vi "串口设备参数设置.vi"(8 "布尔文本.文本":string, 9 "section (optional)":string, 10 "监测项描述":string) -> (2 "布尔":bool=TRUE, 3 "输出簇":T1={"监测项描述:输出"="", "连接方式"=enum."串口", "端口"="", "IP address:"="", "Port:"="", "站号"=19200, "传感器型号"="", "波特率"=19200, "data bits"=8, "停止位"=10, "奇偶校验"=0} {"data bits" min=5 max=8 step=1; "停止位" items=["1.0"=10, "1.5"=15, "2.0"=20]; "奇偶校验" items=["None", "Odd", "Even", "Mark", "Space"]})   [LabVIEW 2016, in "环境动力监测库.lvlib"]
uses:
  <vilib>/Utility/miscctls.llb/LVPointTypeDef.ctl
  <vilib>/Utility/config.llb/NI_LVConfig.lvlib
panel:
  in  "参数配置":bool
  in  "连接方式:":enum16{"串口", "TCP"}(ring)
  in  "IP address:":string
  in  "Port:":string
  in  "data bits":u64=8 caption="数据比特" min=5 max=8 step=1
  in  "波特率":u64=19200
  in  "停止位":u16(ring)=10 items=["1.0"=10, "1.5"=15, "2.0"=20]
  in  "奇偶校验":u16(ring) items=["None", "Odd", "Even", "Mark", "Space"]
  in  "传感器型号:":string(combo)
  in  "输入簇":T1={"监测项描述:输出"="", "连接方式"=enum."串口", "端口"="", "IP address:"="", "Port:"="", "站号"=19200, "传感器型号"="", "波特率"=19200, "data bits"=8, "停止位"=10, "奇偶校验"=0} {"data bits" min=5 max=8 step=1; "停止位" items=["1.0"=10, "1.5"=15, "2.0"=20]; "奇偶校验" items=["None", "Odd", "Even", "Mark", "Space"]}
  in  "站号":u64
  in  "返回":bool
  in  "增加":bool
  in  "端口:":T2(ring)
  in  "监测项描述:":string
  # "基本设置"
  # "如:红外XX"
  # "传感器选择"
  # "端口选择"
  # "站号配置"
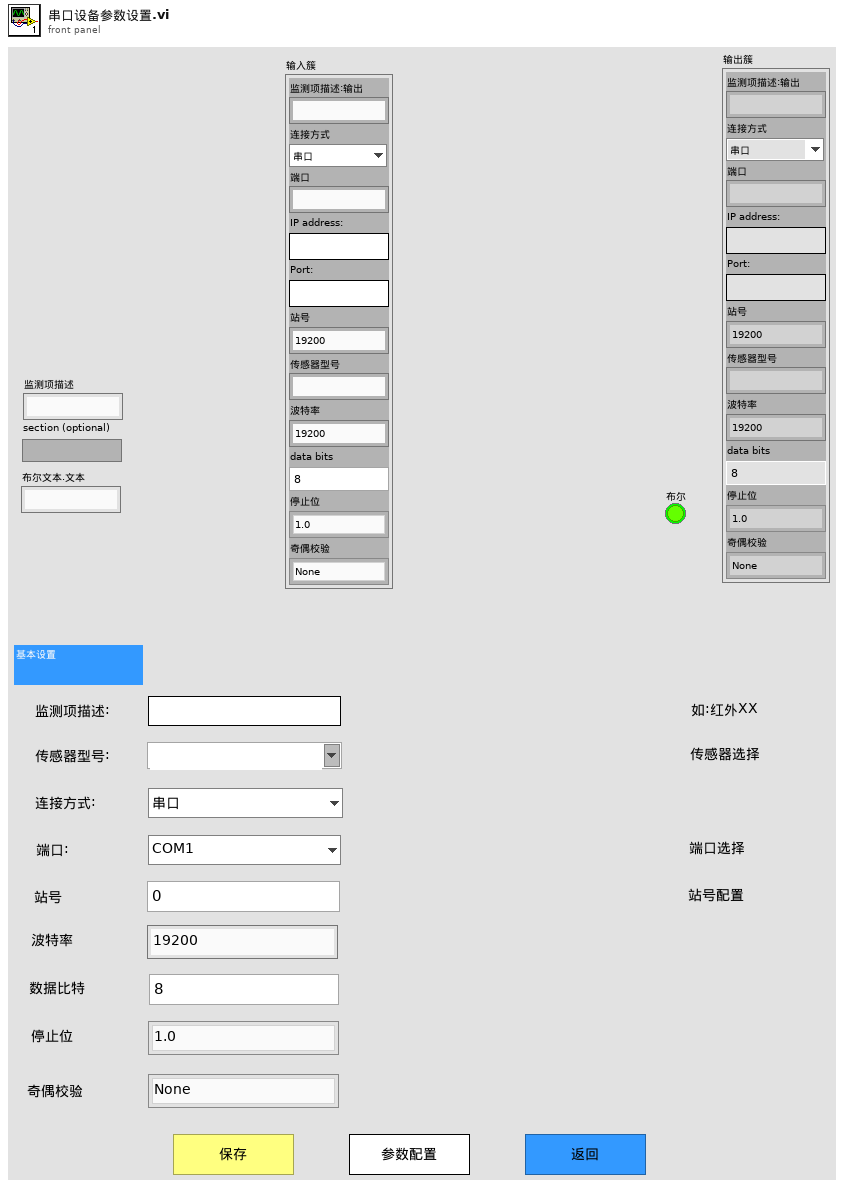
[diagram p1: front panel]
types:
  T1 = cluster{"监测项描述:输出":string, "连接方式":enum16{"串口", "TCP"}, "端口":string, "IP address:":string, "Port:":string, "站号":u64, "传感器型号":string, "波特率":u64, "data bits":u64, "停止位":u16, "奇偶校验":u16}
  T2 = enum16{"COM1", "COM2", "COM3", "COM4", "COM5", "COM6", "COM7", "COM8", "COM9", "COM10", "COM11", "COM12", "COM13", "COM14", "COM15", "COM16", "COM17", "COM18", "COM19", "COM20"}
  T3 = typedef "LVPointTypeDef.ctl" = cluster{"Horizontal":i16, "Vertical":i16}
  T4 = typedef "NI_LVConfig.lvlib/Config Data RefNum.ctl" = refnum<k1>
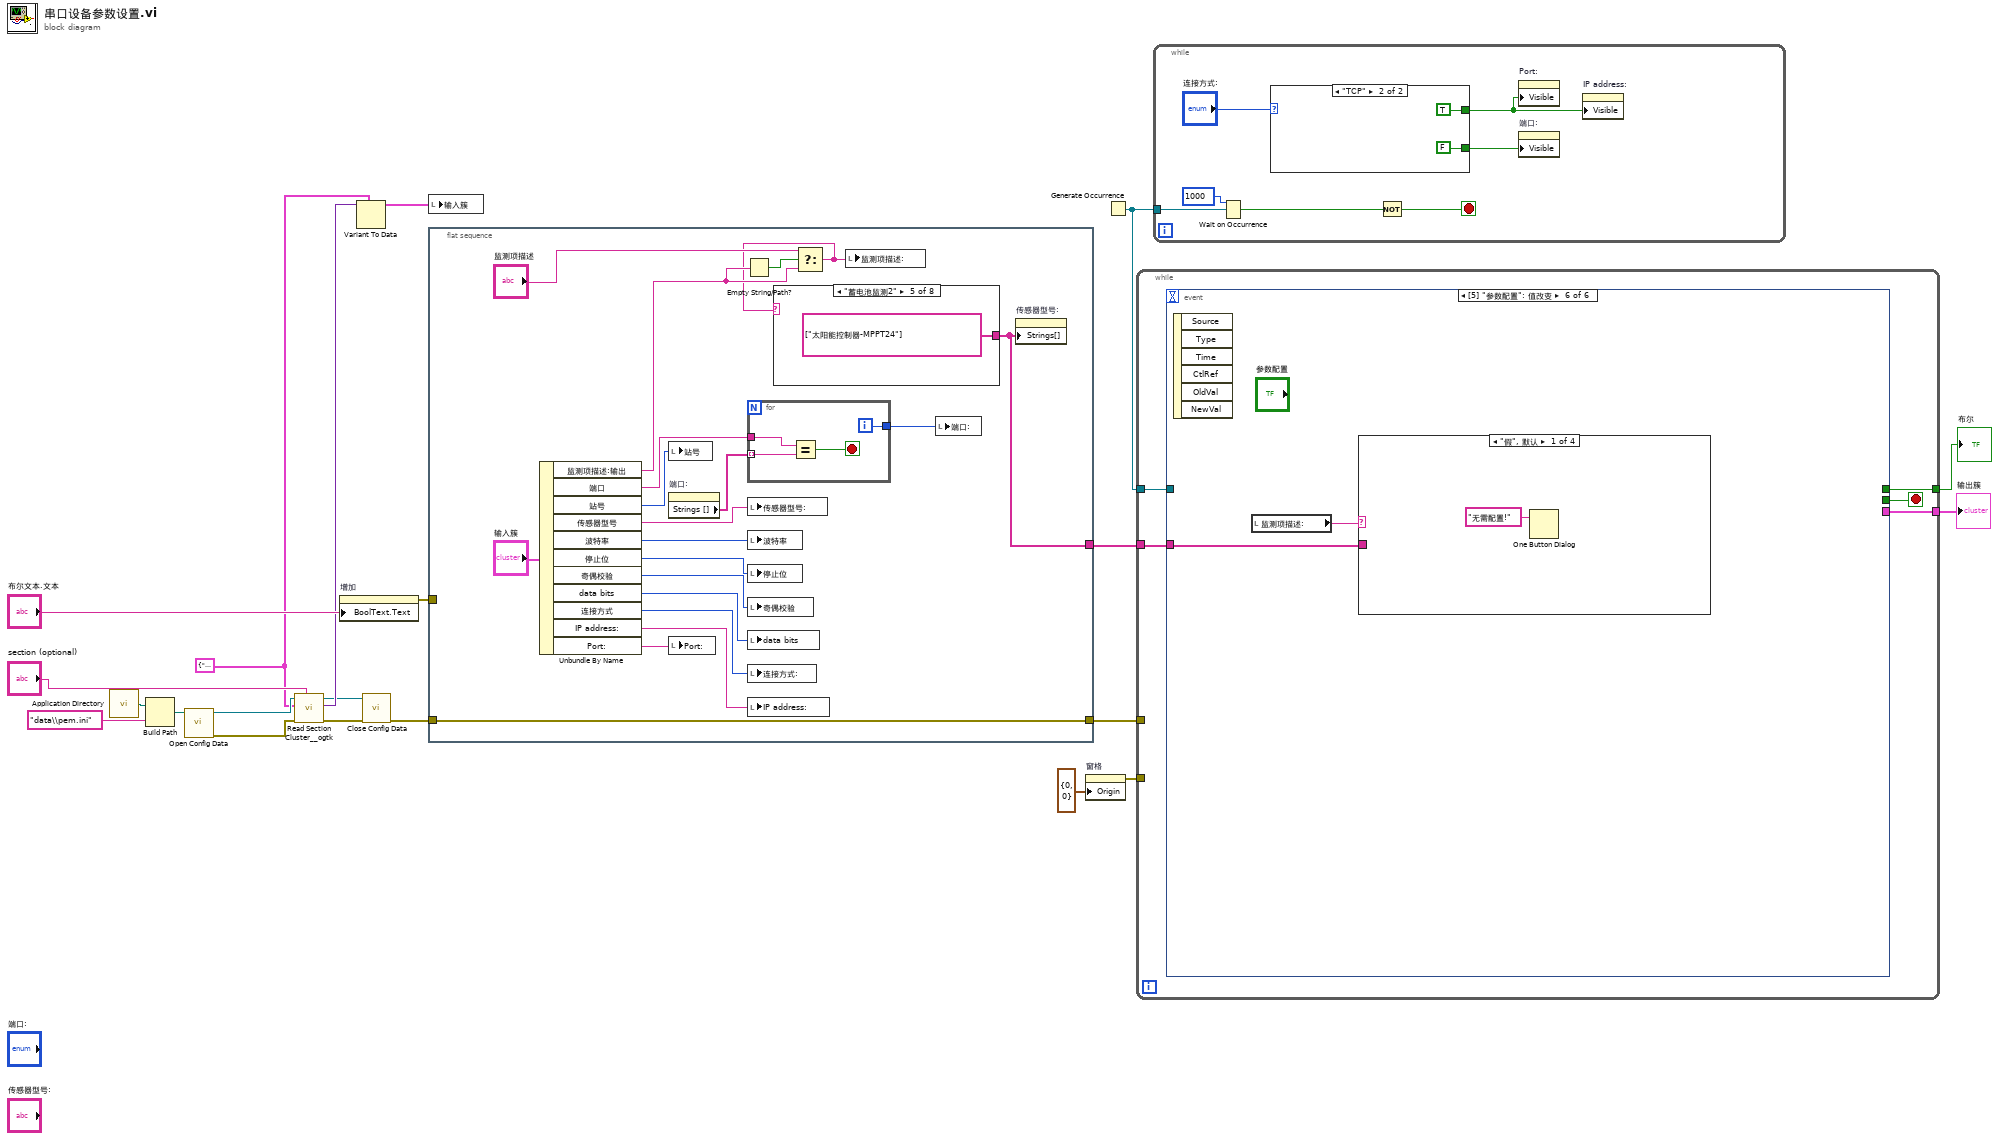
[diagram p0: block diagram]
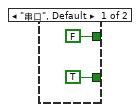
[diagram p2: hidden frame]
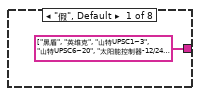
[diagram p3: hidden frame]
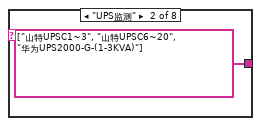
[diagram p4: hidden frame]
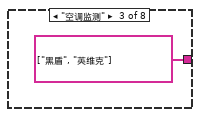
[diagram p5: hidden frame]
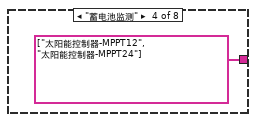
[diagram p6: hidden frame]
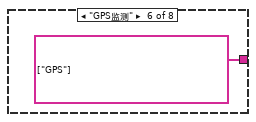
[diagram p7: hidden frame]
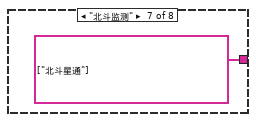
[diagram p8: hidden frame]
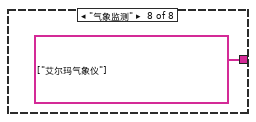
[diagram p9: hidden frame]
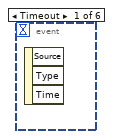
[diagram p10: hidden frame]
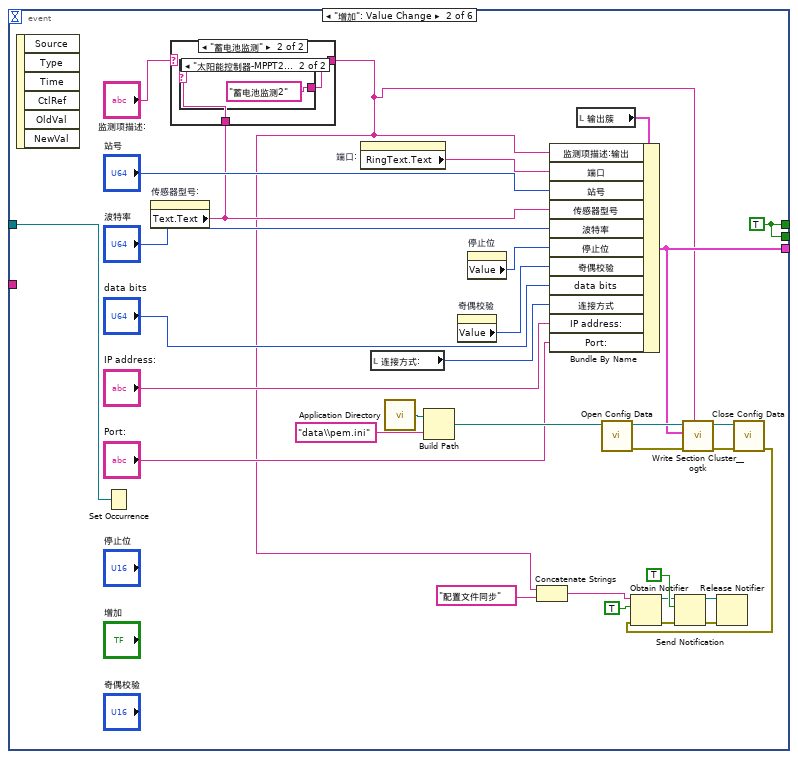
[diagram p11: hidden frame]
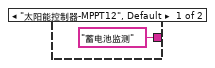
[diagram p13: hidden frame]
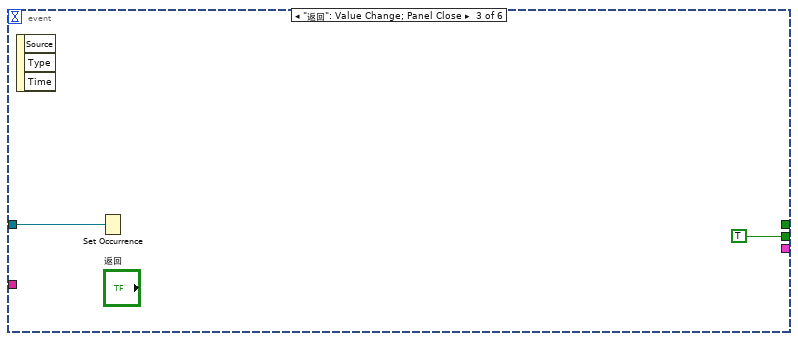
[diagram p14: hidden frame]
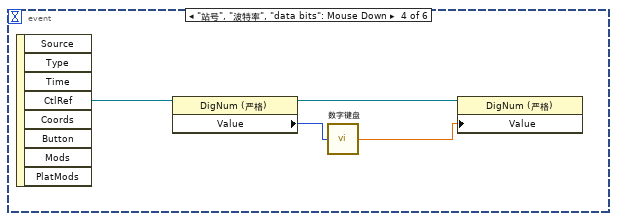
[diagram p15: hidden frame]
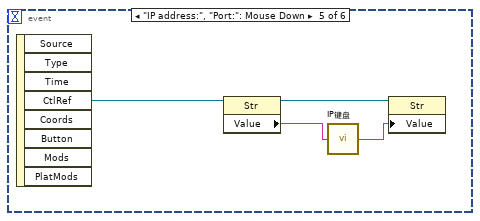
[diagram p16: hidden frame]
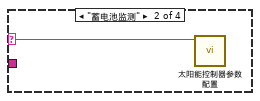
[diagram p17: hidden frame]
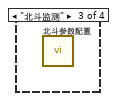
[diagram p18: hidden frame]
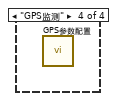
[diagram p19: hidden frame]
diagram:
  w2 = T1 {"监测项描述:输出"="", "连接方式"=enum."串口", "端口"="", "IP address:"="", "Port:"="", "站号"=1, "传感器型号"="", "波特率"=9600, "data bits"=8, "停止位"=10, "奇偶校验"=0} ("输入簇")
  n1 = call <vilib>:"Application Directory.vi"() -> ("Application Directory"=w14:path)
  n2 = Build Path(base path=w14, name or relative path="data\\pem.ini" ("名称或相对路径")) -> (appended path=w15:path)
  n3 = call <vilib>:"Open Config Data.vi"("configuration file path"=w15) -> ("error out"=w16:errorcluster, "refnum"=w17:T4)  [unwired: 8 in, 1 out]
  n4 = call <userlib>:"Read Section Cluster__ogtk.vi"("section (optional)"="section (optional)", "error in (no error)"=w16, "Section Formatted Cluster Type"=w2, "refnum"=w17) -> ("error out"=w9:errorcluster, "Section Formatted Cluster"=w11:variant, "dup refnum"=w10:T4)  [unwired: 3 in, 2 out]
  n5 = property on="增加" class="Bool"("BoolText.Text"="布尔文本.文本") -> (error out=w8:errorcluster)  [unwired: 2 in, 1 out]
  n6 = Variant To Data(type=w2, Variant=w11) -> (data=w3:T1)  [unwired: 1 in, 1 out]
  n7 = call <vilib>:"Close Config Data.vi"("error in (no error)"=w9, "refnum"=w10) -> ("error out"=w7:errorcluster)  [unwired: 8 in, 1 out]
  n8 = local write "输入簇"(w3) -> ()
  n9 = flat-sequence {
    tunnel: w8 -> [_]
    tunnel: w7 -> [w36]
    tunnel: [w36] -> w6
    tunnel: [w22] -> w1
    frame #0 {
      n10 = Unbundle By Name("输入簇") -> ("监测项描述:输出"=w33:string, "端口"=w39:string, "站号"=w24:u64, "传感器型号"=w32:string, "波特率"=w28:u64, "停止位"=w27:u16, "奇偶校验"=w26:u16, "data bits"=w25:u64, "连接方式"=w31:enum16{"串口", "TCP"}, "IP address:"=w30:string, "Port:"=w29:string)
      n11 = local write "站号"(w24) -> ()
      n12 = property on="端口:" class="Enum (严格)"() -> ("Strings []"=w38:string[])  [unwired: 2 in, 2 out]
      n13 = local write "Port:"(w29) -> ()
      n14 = Empty String/Path?(string/path=w33) -> (empty?=w35:bool)
      n15 = for {
        tunnel: w39 -> [w52]
        tunnel: [w50] -> w37
        tunnel: w38 -> [w49] mode=indexing
        i -> [w50]
        stop <- w51 stop-if-true
        n16 = Equal?(x=w52, y=w49) -> (x = y?=w51:bool)
      }
      n17 = local write "传感器型号:"(w32) -> ()
      n18 = local write "波特率"(w28) -> ()
      n19 = local write "停止位"(w27) -> ()
      n20 = local write "奇偶校验"(w26) -> ()
      n21 = local write "data bits"(w25) -> ()
      n22 = local write "连接方式:"(w31) -> ()
      n23 = local write "IP address:"(w30) -> ()
      n24 = Select(t="监测项描述", s=w35, f=w33) -> (s? t:f=w23:string)
      n25 = case shown="\"蓄电池监测2\"" w23 {
        tunnel: [string[] ["黑盾", "英维克", "山特UPSC1~3", "山特UPSC6~20", "太阳能控制器-12/24", "华为UPS2000-G-(1-3KVA)"] ("字符串[]") string[] ["山特UPSC1~3", "山特UPSC6~20", "华为UPS2000-G-(1-3KVA)"] ("字符串[]") string[] ["黑盾", "英维克"] ("字符串[]") string[] ["太阳能控制器-MPPT12", "太阳能控制器-MPPT24"] ("字符串[]") string[] ["太阳能控制器-MPPT24"] ("字符串[]") string[] ["GPS"] ("字符串[]") string[] ["北斗星通"] ("字符串[]") string[] ["艾尔玛气象仪"] ("字符串[]")] -> w22
        frame "假", Default {
        }
        frame "UPS监测" {
        }
        frame "空调监测" {
        }
        frame "蓄电池监测" {
        }
        frame "蓄电池监测2" {
        }
        frame "GPS监测" {
        }
        frame "北斗监测" {
        }
        frame "气象监测" {
        }
      }
      n26 = local write "监测项描述:"(w23) -> ()
      n27 = local write "端口:"(w37) -> ()
      n28 = property on="传感器型号:" class="CmbBox"("Strings[]"=w22) -> ()  [unwired: 2 in, 2 out]
    }
  }
  n29 = property on="窗格" class="Pane"("Origin"=T3 {"Horizontal"=0, "Vertical"=0} ("原点")) -> (error out=w21:errorcluster)  [unwired: 2 in, 1 out]
  n30 = Generate Occurrence() -> (w4:refnum<k4>)
  n31 = while {
    tunnel: w21 -> [_]
    tunnel: [w57] -> w5
    tunnel: [w55] -> w19
    tunnel: w6 -> [_]
    tunnel: w4 -> [w54]
    tunnel: w1 -> [w53]
    stop <- w56 stop-if-true
    n32 = event shown="[5] \"参数配置\": 值改变" {
      selector: _ -> [_ _ _ _ _ _]
      dyn-events: _ -> [_ _ _ _ _ _]
      timeout: _ -> [_ _ _ _ _ _]
      tunnel: [_ w82 _ _ _ _] -> w57
      tunnel: [_ w81 TRUE _ _ _] -> w56
      tunnel: [_ w81 _ _ _ _] -> w55
      tunnel: w54 -> [_ w78 w95 _ _ _]
      tunnel: w53 -> [_ _ _ _ _ w105]
      event Timeout {
        n33 = event-data() -> ()  [unwired: 1 in, 3 out]
      }
      event "增加": Value Change {
        w81 = TRUE
        n34 = event-data() -> ()  [unwired: 1 in, 6 out]
        n35 = Set Occurrence(w78) -> ()
        n36 = property on="传感器型号:" class="CmbBox"() -> ("Text.Text"=w59:string)  [unwired: 2 in, 2 out]
        n37 = case shown="\"蓄电池监测\"" "监测项描述:" {
          selector: "监测项描述:" -> [w90 _]
          tunnel: w59 -> [_ w92]
          tunnel: [w90 w91] -> w58
          frame "假", Default {
          }
          frame "蓄电池监测" {
            n38 = case shown="\"太阳能控制器-MPPT24\"" w92 {
              tunnel: ["蓄电池监测" ("section (optional)") "蓄电池监测2" ("section (optional)")] -> w91
              frame "太阳能控制器-MPPT12", Default {
              }
              frame "太阳能控制器-MPPT24" {
              }
            }
          }
        }
        n39 = property on="端口:" class="Enum (严格)"() -> ("RingText.Text"=w80:string)  [unwired: 2 in, 2 out]
        n40 = local read "连接方式:"() -> (w70:enum16{"串口", "TCP"})
        n41 = call <vilib>:"Application Directory.vi"() -> ("Application Directory"=w86:path)
        n42 = Build Path(base path=w86, name or relative path="data\\pem.ini" ("名称或相对路径")) -> (appended path=w87:path)
        n43 = property on="奇偶校验" class="Ring (严格)"() -> ("Value"=w79:u16)  [unwired: 2 in, 2 out]
        n44 = property on="停止位" class="Ring (严格)"() -> ("Value"=w75:u16)  [unwired: 2 in, 2 out]
        n45 = Concatenate Strings(w58, "配置文件同步" ("名称（未命名）")) -> (w61:string)
        n46 = local read "输出簇"() -> (w77:T1)
        n47 = Bundle By Name(cluster=w77, "监测项描述:输出"=w58, "端口"=w80, "站号"="站号", "传感器型号"=w59, "波特率"="波特率", "停止位"=w75, "奇偶校验"=w79, "data bits"="data bits", "连接方式"=w70, "IP address:"="IP address:", "Port:"="Port:") -> (w82:T1)
        n48 = call <vilib>:"Open Config Data.vi"("configuration file path"=w87) -> ("error out"=w88:errorcluster, "refnum"=w89:T4)  [unwired: 8 in, 1 out]
        n49 = call <userlib>:"Write Section Cluster__ogtk.vi"("section (optional)"=w58, "error in (no error)"=w88, "Section Formatted Cluster"=w82, "refnum"=w89) -> ("error out"=w83:errorcluster, "dup refnum"=w84:T4)  [unwired: 6 in]
        n50 = call <vilib>:"Close Config Data.vi"("error in (no error)"=w83, "refnum"=w84) -> ("error out"=w66:errorcluster)  [unwired: 8 in, 1 out]
        n51 = Obtain Notifier(name (unnamed)=w61, notification data type=TRUE, error in (no error)=w66) -> (notifier out=w65:refnum<notifier>, error out=w67:errorcluster)  [unwired: 1 in, 1 out]
        n52 = Send Notification(notification=TRUE ("通知"), notifier=w65, error in (no error)=w67) -> (notifier out=w64:refnum<notifier>, error out=w63:errorcluster)
        n53 = Release Notifier(notifier=w64, error in (no error)=w63) -> ()  [unwired: 1 in, 3 out]
      }
      event "返回": Value Change; Panel Close {
        n54 = event-data() -> ()  [unwired: 1 in, 3 out]
        n55 = Set Occurrence(w95) -> ()
      }
      event "站号", "波特率", "data bits": Mouse Down {
        n56 = event-data() -> ("CtlRef"=w100:refnum<vi>)  [unwired: 1 in, 7 out]
        n57 = property class="DigNum (严格)"(reference=w100) -> (reference out=w98:refnum<vi>, "Value"=w99:u64)  [unwired: 1 in, 1 out]
        n58 = call "数字键盘.vi"("OldNumber"=w99) -> ("NewNumber"=w97:sgl)
        n59 = property class="DigNum (严格)"(reference=w98, "Value"=w97) -> ()  [unwired: 1 in, 2 out]
      }
      event "IP address:", "Port:": Mouse Down {
        n60 = event-data() -> ("CtlRef"=w104:refnum<vi>)  [unwired: 1 in, 7 out]
        n61 = property class="Str"(reference=w104) -> (reference out=w103:refnum<vi>, "Value"=w102:string)  [unwired: 1 in, 1 out]
        n62 = call "IP键盘.vi"("OldNumber"=w102) -> ("NewNumber"=w101:string)
        n63 = property class="Str"(reference=w103, "Value"=w101) -> ()  [unwired: 1 in, 2 out]
      }
      event "参数配置": Value Change {
        n64 = event-data() -> ()  [unwired: 1 in, 6 out]
        n65 = local read "监测项描述:"() -> (w106:string)
        n66 = case shown="\"假\", 默认" w106 {
          selector: w106 -> [_ w108 _ _]
          tunnel: w105 -> [_ _ _ _]
          frame "假", Default {
            n67 = One Button Dialog(message="无需配置!" ("消息")) -> ()  [unwired: 1 in, 1 out]
          }
          frame "蓄电池监测" {
            n68 = call "太阳能控制器参数配置.vi"("监测项描述"=w108) -> ()  [unwired: 11 in]
          }
          frame "北斗监测" {
            n69 = call "北斗参数配置.vi"() -> ()  [unwired: 12 in]
          }
          frame "GPS监测" {
            n70 = call "GPS参数配置.vi"() -> ()  [unwired: 12 in]
          }
        }
      }
    }
  }
  "输出簇" <- w5
  "布尔" <- w19
  n71 = while {
    tunnel: w4 -> [w115]
    stop <- w112 stop-if-true
    n72 = Wait on Occurrence(2:w115, 3:1000 ("毫秒超时(-1)")) -> (0:w113:bool)  [unwired: 1 in]
    n73 = case shown="\"TCP\"" "连接方式:" {
      tunnel: [TRUE FALSE] -> w110
      tunnel: [FALSE TRUE] -> w109
      frame "串口", Default {
      }
      frame "TCP" {
      }
    }
    n74 = Not(x=w113) -> (.not. x?=w112:bool)
    n75 = property on="Port:" class="Str"("Visible"=w109) -> ()  [unwired: 2 in, 2 out]
    n76 = property on="端口:" class="Enum (严格)"("Visible"=w110) -> ()  [unwired: 2 in, 2 out]
    n77 = property on="IP address:" class="Str"("Visible"=w109) -> ()  [unwired: 2 in, 2 out]
  }
